vi "vision target evaluator.vi"(1 "Area":dbl, 2 "Height":dbl, 3 "Width":dbl) -> (0 "result":bool)   [LabVIEW 2015]
panel:
  out "Area In Range?":bool
  out "Height In Range?":bool
  out "Width In Range?":bool
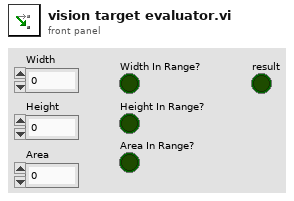
[diagram p1: front panel]
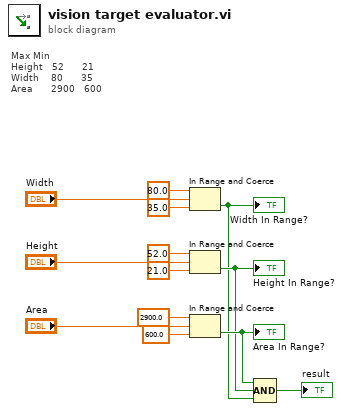
[diagram p0: block diagram]
diagram:
  # "Max\tMin\nHeight\t  52\t     21\nWidth    80     \t35\nArea\t     2900\t  600"
  n1 = In Range and Coerce(upper limit=80.0, x="Width", lower limit=35.0) -> (In Range?=w2:bool)  [unwired: 1 out]
  "Width In Range?" <- w2
  n2 = In Range and Coerce(upper limit=52.0, x="Height", lower limit=21.0) -> (In Range?=w3:bool)  [unwired: 1 out]
  "Height In Range?" <- w3
  n3 = In Range and Coerce(upper limit=2900.0, x="Area", lower limit=600.0) -> (In Range?=w4:bool)  [unwired: 1 out]
  "Area In Range?" <- w4
  n4 = Compound Arithmetic op=AND(w4, w3, w2) -> (→"result":bool)
